vi "Write String Table.vi"(0 "Report Ref In":T1, 1 "Start Row Index":i32, 2 "Start Column Index":i32, 3 "error in (no error)":errorcluster, 4 "Input Range":string[][](array[string])) -> (5 "Report Ref Out":T1, 6 "error out":errorcluster)   [LabVIEW 2026, in "XCel Report Engine.lvlib"]
uses:
  XCel Report Engine.lvlib
  Controls/Report Ref.ctl
  C:/Users/m.santucci/Documents/ChatGPT/LV_REPORT_ENGINE/.net/src/XCelReportEngine/bin/Release/net48/XCelReportEngine.dll
  .net/src/XCelReportEngine/bin/Release/net48/XCelReportEngine.dll
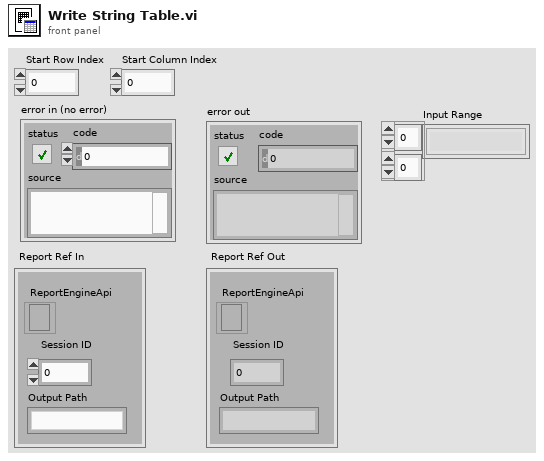
[diagram p1: front panel]
types:
  T1 = typedef "XCel Report Engine.lvlib/Report Ref.ctl" = cluster{"Session ID":i32, "Output Path":string, "ReportEngineApi":refnum<k24>}
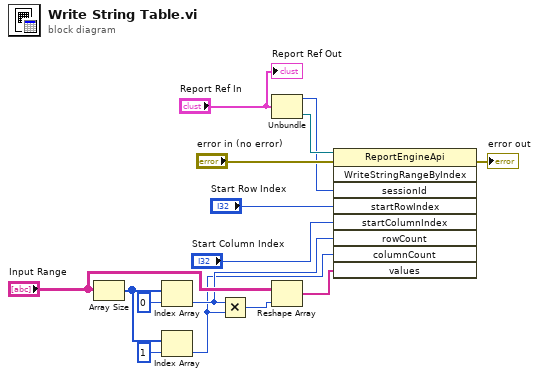
[diagram p0: block diagram]
diagram:
  n1 = Array Size(array="Input Range") -> (size(s)=w5:i32[])
  n2 = Index Array(array=w5, index=0) -> (element=w3:i32)
  n3 = Index Array(array=w5, index=1) -> (element=w2:i32)
  n4 = Multiply(x=w3, y=w2) -> (x*y=w1:i32)
  n5 = Unbundle("Report Ref In") -> ("Session ID"=w11:i32, "ReportEngineApi"=w14:refnum<k24>)  [unwired: 1 out]
  n6 = Reshape Array("Input Range", w1) -> (w7:string[])
  n7 = invoke class="ReportEngineApi" method="WriteStringRangeByIndex"(reference=w14, error in="error in (no error)", "sessionId"=w11, "startRowIndex"="Start Row Index", "startColumnIndex"="Start Column Index", "rowCount"=w3, "columnCount"=w2, "values"=w7) -> (error out=→"error out":errorcluster)  [unwired: 1 in, 8 out]
  "Report Ref Out" <- "Report Ref In"
